vi "EMV PI Controller Estimate.vi"(8 "error in (no error)":errorcluster, 11 "Mixing Valve.MixValveAbsoluteStepPosition (0x400B)":i16) -> (0 "error out":errorcluster, 3 "PI End of Flow Detection":bool)   [LabVIEW 2020]
panel:
  out "slope":dbl
  out "standard deviation":dbl format="%0.2f"
  out "Waveform Chart":dbl(graph)
  out "Step Position History":dbl[](array[numeric])
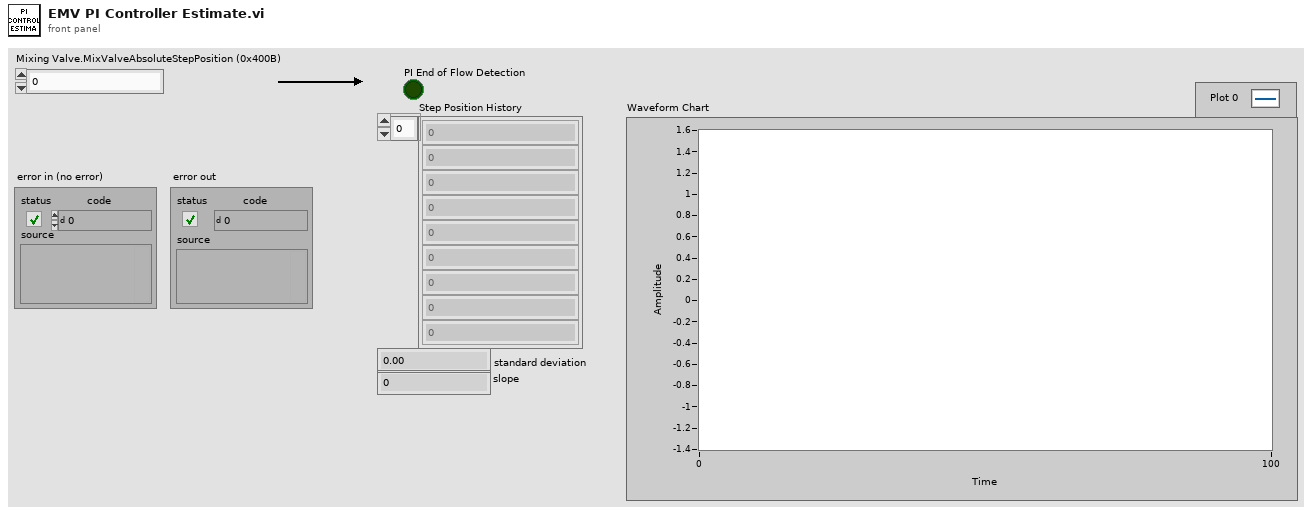
[diagram p1: front panel]
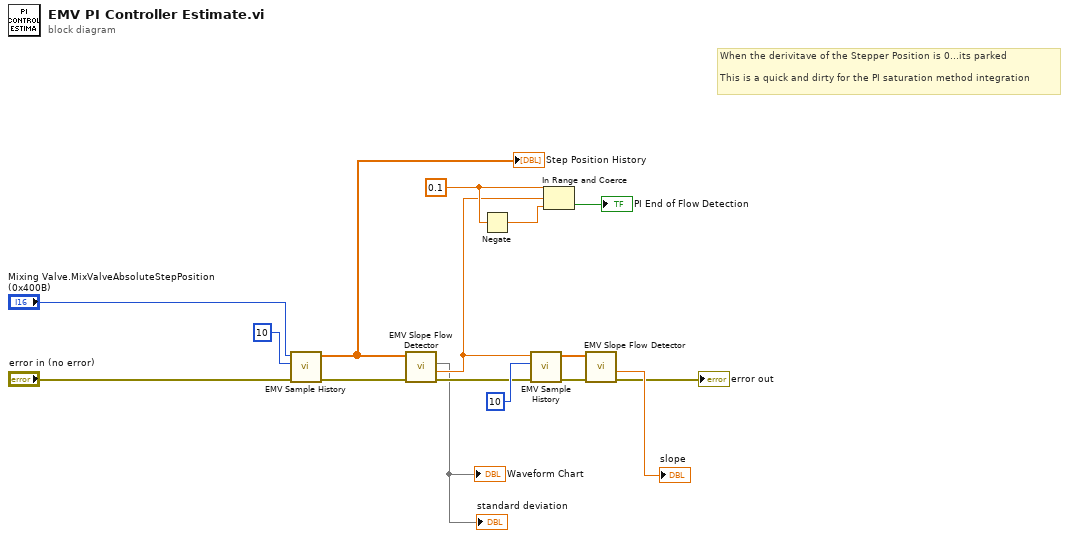
[diagram p0: block diagram]
diagram:
  w11 = 0.1 ("upper limit")
  # "When the derivitave of the Stepper Position is 0...its parked\n\nThis is a quick and dirty for the PI saturation method integration"
  n1 = call "EMV Sample History.vi"("error in (no error)"="error in (no error)", "length"=10, "T6 Temp"="Mixing Valve.MixValveAbsoluteStepPosition (0x400B)") -> ("error out"=w16:errorcluster, "T6 History"=w15:dbl[])  [unwired: 7 in]
  "Step Position History" <- w15
  n2 = call "EMV Slope Flow Detector.vi"("error in (no error)"=w16, "Current T6 Temperatures in"=w15) -> ("error out"=w6:errorcluster, "slope"=w7:dbl, 2:→"Waveform Chart" →"standard deviation")  [unwired: 6 in, 1 out]
  n3 = Negate(x=w11) -> (-x=w12:dbl)
  n4 = call "EMV Sample History.vi"("error in (no error)"=w6, "length"=10, "T6 Temp"=w7) -> ("error out"=w5:errorcluster, "T6 History"=w4:dbl[])  [unwired: 7 in]
  n5 = In Range and Coerce(upper limit=w11, x=w7, lower limit=w12) -> (In Range?=→"PI End of Flow Detection":bool)  [unwired: 1 out]
  n6 = call "EMV Slope Flow Detector.vi"("error in (no error)"=w5, "Current T6 Temperatures in"=w4) -> ("error out"=→"error out":errorcluster, "slope"=→"slope":dbl)  [unwired: 7 in, 1 out]
